vi "VI-Add Child To Factory.vi"(0 "LVClassLibrary in":refnum<vi>, 2 "Parent":refnum<vi>, 11 "error in (no error)":errorcluster) -> (4 "LVClassLibrary out":refnum<vi>, 15 "error out":errorcluster)   [LabVIEW 2020]
uses:
  <vilib>/Utility/traverseref.llb/TRef TravTarget.ctl
  <vilib>/Utility/traverseref.llb/VI Scripting - Traverse.lvlib
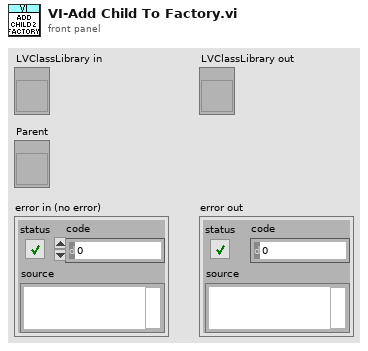
[diagram p1: front panel]
types:
  T1 = typedef "TRef TravTarget.ctl" = enum16{"FP", "BD", "Other"}
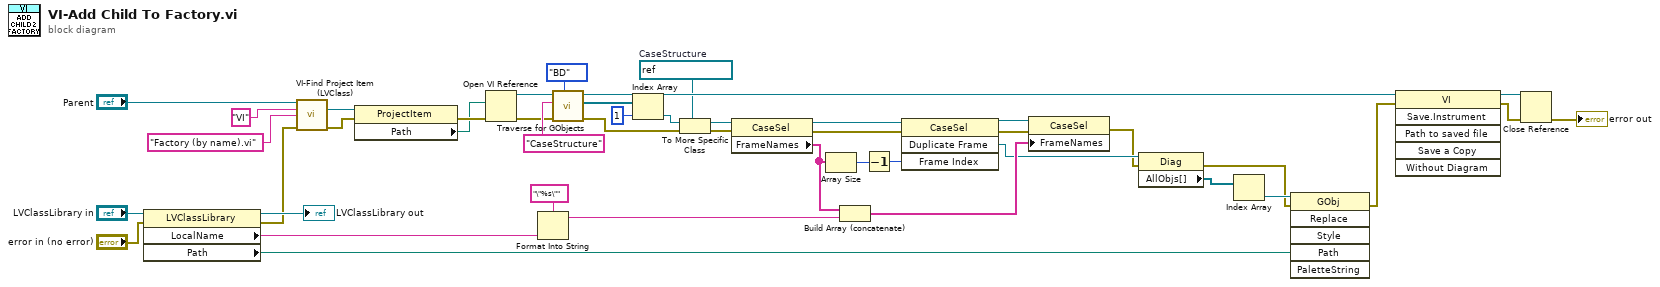
[diagram p0: block diagram]
diagram:
  w22 = refnum<vi> refnum  # CaseStructure
  n1 = property class="LVClassLibrary"(reference="LVClassLibrary in", error in="error in (no error)") -> (reference out=→"LVClassLibrary out":refnum<vi>, error out=w18:errorcluster, "LocalName"=w23:string, "Path"=w3:path)
  n2 = call "VI-Find Project Item (LVClass).vi"("LVClassLibrary Refnum"="Parent", "Type"="VI", "Name"="Factory (by name).vi" ("name or relative path"), "error in (no error)"=w18) -> ("ProjectItem"=w39:refnum<vi>, "error out"=w40:errorcluster)  [unwired: 9 in, 1 out]
  n3 = property class="ProjectItem"(reference=w39, error in=w40) -> (error out=w38:errorcluster, "Path"=w37:path)  [unwired: 1 out]
  n4 = Open VI Reference(vi path=w37, error in (no error)=w38) -> (vi reference=w26:refnum<vi>, error out=w27:errorcluster)  [unwired: 4 in]
  n5 = Format Into String(format string="\"%s\"", w23) -> (resulting string=w36:string)  [unwired: 2 in, 1 out]
  n6 = call <vilib>:"Traverse for GObjects.vi"("Traverse Target"=TRef_TravTarget."BD", "error in (no error)"=w27, "Class Name"="CaseStructure", "VI Refnum"=w26) -> ("error out"=w31:errorcluster, "References"=w33:refnum<vi>[], "dup VI Refnum"=w30:refnum<vi>)  [unwired: 4 in, 1 out]
  n7 = Index Array(array=w33, index=1) -> (element=w20:refnum<vi>)
  n8 = To More Specific Class(target class=w22, reference=w20, error in=w31) -> (specific class reference=w21:refnum<vi>, error out=w15:errorcluster)
  n9 = property class="CaseSel"(reference=w21, error in=w15) -> (reference out=w16:refnum<vi>, error out=w14:errorcluster, "FrameNames"=w10:string[])
  n10 = Array Size(array=w10) -> (size(s)=w13:i32)
  n11 = Build Array (concatenate)(w10, w36) -> (w9:string[])
  n12 = Decrement(x=w13) -> (x-1=w12:i32)
  n13 = invoke class="CaseSel" method="Duplicate Frame"(reference=w16, error in=w14, "Frame Index"=w12) -> (reference out=w11:refnum<vi>, error out=w7:errorcluster, "Duplicate Frame"=w6:refnum<vi>)  [unwired: 1 in, 1 out]
  n14 = property class="CaseSel"(reference=w11, error in=w7, "FrameNames"=w9) -> (error out=w5:errorcluster)  [unwired: 1 out]
  n15 = property class="Diag"(reference=w6, error in=w5) -> (error out=w2:errorcluster, "AllObjs[]"=w8:refnum<vi>[])  [unwired: 1 out]
  n16 = Index Array(array=w8) -> (element=w4:refnum<vi>)  [unwired: 1 in]
  n17 = invoke class="GObj" method="Replace"(reference=w4, error in=w2, "Path"=w3) -> (error out=w1:errorcluster)  [unwired: 3 in, 5 out]
  n18 = invoke class="VI" method="Save.Instrument"(reference=w30, error in=w1) -> (reference out=w32:refnum<vi>, error out=w34:errorcluster)  [unwired: 4 in, 4 out]
  n19 = Close Reference(reference=w32, error in (no error)=w34) -> (error out=→"error out":errorcluster)
